vi "ZiptItup.vi"(9 "Folder to zip":path, 11 "Zip file":path) -> (0 "error out":errorcluster, 3 "Generated Zip File":path)   [LabVIEW 2022 SP3]
panel:
  out "All Files in Dir":path[](array[path])
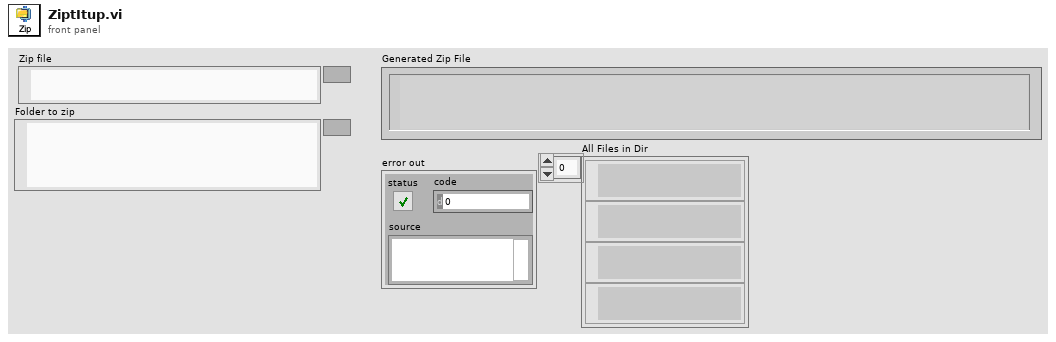
[diagram p1: front panel]
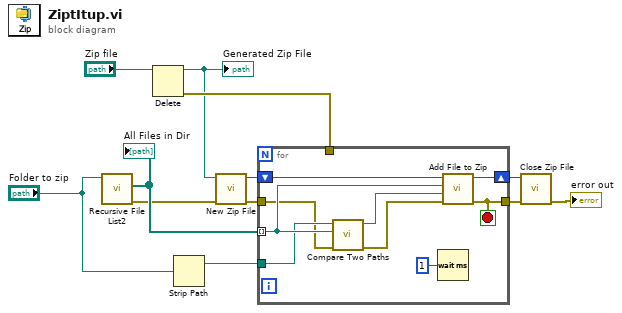
[diagram p0: block diagram]
diagram:
  n1 = call "Recursive File List2.vi"("Folder Path"="Folder to zip") -> ("error out"=w6:errorcluster, "All Files in Dir"=w7:path[])  [unwired: 6 in, 3 out]
  "All Files in Dir" <- w7
  n2 = Delete(path (use dialog)="Zip file") -> (deleted path=w9:path, error out=w11:errorcluster)  [unwired: 4 in, 1 out]
  "Generated Zip File" <- w9
  n3 = Strip Path(path="Folder to zip") -> (stripped path=w10:path)  [unwired: 1 out]
  n4 = call <vilib>:"New Zip File.vi"("error in (no error)"=w6, "target"=w9) -> ("error out"=w3:errorcluster, "zip file out"=w2:i64)  [unwired: 1 in, 3 out]
  n5 = for {
    tunnel: w7 -> [w18] mode=indexing
    tunnel: w3 -> [w15]
    tunnel: [w19] -> w4
    shift-right: [w20] -> w5
    shift-left: w2 -> [w21]
    tunnel: w10 -> [w17]
    tunnel: w11 -> [_]
    stop <- w19 stop-if-true
    n6 = call <vilib>:"Compare Two Paths.vi"("error in (no error)"=w15, "Path 2"=w18, "Path 1"=w17) -> ("error out"=w14:errorcluster, "Relative Path from 1 to 2"=w16:path)  [unwired: 5 in, 2 out]
    n7 = Wait (ms)(milliseconds to wait=u32 1) -> ()  [unwired: 1 out]
    n8 = call <vilib>:"Add File to Zip.vi"("error in (no error)"=w14, "destination path in zip"=w16, "source file path"=w18, "zip file in"=w21) -> ("error out"=w19:errorcluster, "zip file out"=w20:i64)  [unwired: 6 out]
  }
  n9 = call <vilib>:"Close Zip File.vi"("error in (no error)"=w4, "zip file in"=w5) -> ("error out"=→"error out":errorcluster)  [unwired: 1 in, 4 out]
